vi "PPL_SIM_SIM_Execute.vi"(6 "FPGA_Time_Seconds":dbl, 8 "error in (no error)":errorcluster) -> (0 "error out":errorcluster)   [LabVIEW 2019]
uses:
  <vilib>/Rock Robotics/WPI/ThirdParty/JAS_Junk/TrajLib/Enum/DCMOTOR_TYPES_ENUM.ctl
  <vilib>/Rock Robotics/WPI/ThirdParty/JAS_Junk/TrajLib/Enum/DIFF_DRIVE_ToughBoxMini_GearChoice_ENUM.ctl
  <vilib>/Rock Robotics/WPI/ThirdParty/JAS_Junk/TrajLib/Enum/DIFF_DRIVE_TRAIN_SIM_STATE_ENUM.ctl
  <vilib>/Rock Robotics/WPI/ThirdParty/JAS_Junk/TrajLib/Rotation2d_CreateAngle.vi
  <vilib>/Rock Robotics/WPI/ThirdParty/JAS_Junk/TrajLib/Translation2d_Create.vi
  <vilib>/Rock Robotics/WPI/ThirdParty/JAS_Junk/TrajLib/BatterySim_CalculateLoadedBatteryVoltage.vi
  PPL_SIM_SIM_Globals.vi
  <vilib>/Rock Robotics/WPI/ThirdParty/JAS_Junk/TrajLib/Trajectory_Library.lvlib
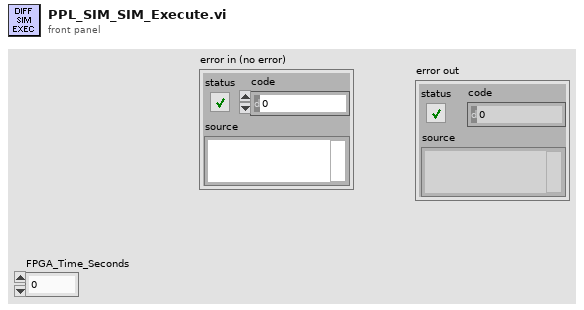
[diagram p1: front panel]
types:
  T1 = typedef "Trajectory_Library.lvlib/DIFF_DRIVE_TRAIN_SIM_STATE_ENUM.ctl" = enum16{"X_POS", "Y_POS", "HEADING", "LEFT_VEL", "RIGHT_VEL", "LEFT_DIST", "RIGHT_DIST"}
  T2 = typedef "Trajectory_Library.lvlib/DIFF_DRIVE_ToughBoxMini_GearChoice_ENUM.ctl" = enum16{"Ratio_12_75", "Ratio_10_71", "Ratio_8_45", "Ratio_7_31", "Ratio_5_95"}
  T3 = typedef "Trajectory_Library.lvlib/DCMOTOR_TYPES_ENUM.ctl" = enum16{"CIM", "AndyMark 9015", "Andy Mark RS 775 125", "Bag", "BaneBots RS 550", "BaneBots RS 775", "Falcon 500", "Mini CIM", "NEO", "NEO 550", "Romi BuiltIn", "Vex 775 Pro", "Snow Blower AM 2235A", "Bosch Seat AM 3493"}
  T4 = cluster{"Diff Motor Device Index":i32, "Wheel Encoder Device Index":i32, "Wheel DistPerzcount":dbl}[]
  T5 = cluster{"Diff Motor Device Index":i32, "Wheel Encoder Device Index":i32, "Wheel DistPerzcount":dbl}
  T6 = typedef "Trajectory_Library.lvlib/POSE2D.ctl" = cluster{"TRANSLATION":T7, "ROTATION":T8}
  T7 = typedef "Trajectory_Library.lvlib/TRANSLATION2D.ctl" = cluster{"X":dbl, "Y":dbl}
  T8 = typedef "Trajectory_Library.lvlib/ROTATION2D.ctl" = cluster{"VALUE":dbl, "COS":dbl, "SIN":dbl}
  T9 = typedef "Trajectory_Library.lvlib/DIFF_DRIVE_ODOM2.ctl" = cluster{"M_POSE_Meters":T6, "M_GyroOffset":T8, "M_PrevAngle":T8, "M_PrevLeftDist_M":dbl, "M_PrevRightDist_M":dbl, "M_InitLeftDist_M":dbl, "M_InitRightDist_M":dbl}
  T10 = typedef "Trajectory_Library.lvlib/DIFF_DRIVE_SIM_SIMULATION_PARAMS.ctl" = cluster{"X Pos Meas Std Dev M":dbl, "Y Pos Meas Std Dev M":dbl, "Heading Meas Std Dev Rad":dbl, "Left Vel Meas Std Dev M/S":dbl, "Right Vel Meas Std Dev M/S":dbl, "Left Pos Meas Std Dev M":dbl, "Right Pos Meas Std Dev M":dbl}
  T11 = typedef "Trajectory_Library.lvlib/DIFF_DRIVE_SIM_MODEL_PARAMS.CTL" = cluster{"TracWidth_M":dbl, "WheelRadius_M":dbl, "Gearing":dbl, "Mass kg":dbl, "MOI kgm2":dbl, "DCMOTOR_TYPES":T3, "Num Motors":i32}
  T12 = typedef "Trajectory_Library.lvlib/DIFF_DRIVE_TRAIN_SIM.ctl" = cluster{"m_Plant":T13, "m_X":T14, "m_Y":T14, "m_U":T14, "MeasureStdDev":T14, "m_Motor":T15, "m_OriginalGearing":dbl, "m_CurrentGearing":dbl, "m_WheelRadius_M":dbl, "m_RB":dbl}
  T13 = typedef "Trajectory_Library.lvlib/LINEAR_SYSTEM.ctl" = cluster{"m_A":T14, "m_B":T14, "m_C":T14, "m_D":T14, "States":i32, "Inputs":i32, "Outputs":i32}
  T14 = typedef "NI_Matrix.lvlib/RealMatrix.ctl" = dbl[][]
  T15 = typedef "Trajectory_Library.lvlib/DCMOTOR.CTL" = cluster{"nominalVoltage_Volts":dbl, "StallTorque_NM":dbl, "StallCurrent_Amps":dbl, "FreeCurrent_Amps":dbl, "FreeSpeed_RadPerSec":dbl, "R_Ohms":dbl, "KvINV_RadPerSecPerVolt":dbl, "Kt_NMPerAmp":dbl, "L_H":dbl, "Jr_KgM2":dbl}
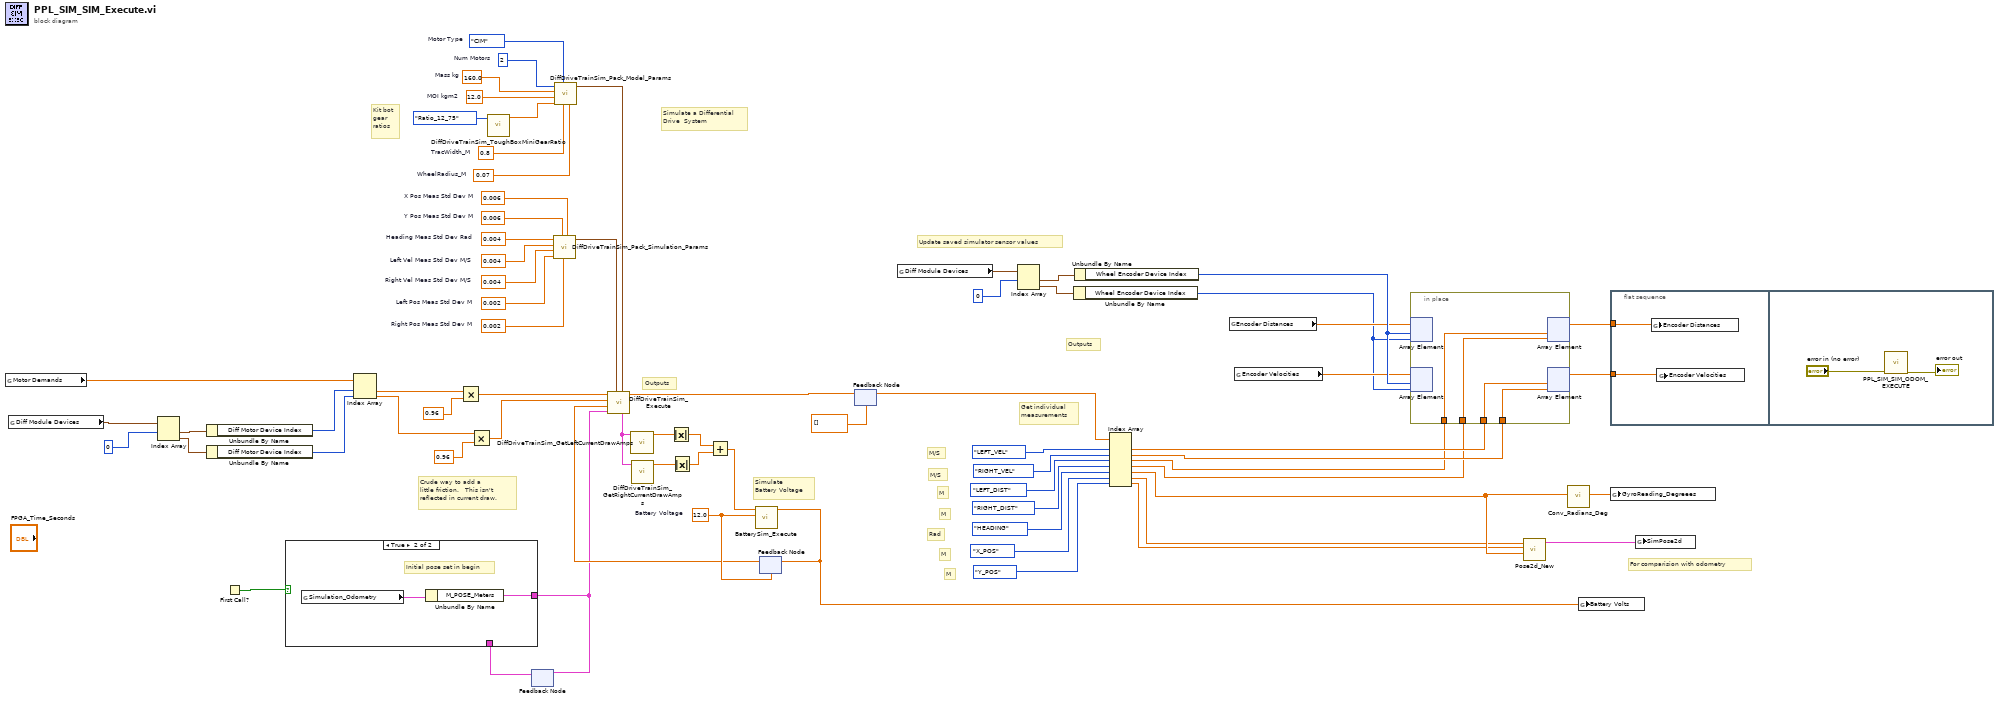
[diagram p0: block diagram]
diagram:
  w57 = 160.0  # Mass kg
  w58 = 12.0  # MOI kgm2
  w59 = 0.8  # TracWidth_M
  w60 = 0.07  # WheelRadius_M
  w61 = 0.004  # Heading Meas Std Dev Rad
  w62 = 0.004  # Left Vel Meas Std Dev M/S
  w63 = 0.004  # Right Vel Meas Std Dev M/S
  w64 = 0.002  # Left Pos Meas Std Dev M
  w65 = 0.006  # Y Pos Meas Std Dev M
  w66 = 0.002  # Right Pos Meas Std Dev M
  w67 = 0.006  # X Pos Meas Std Dev M
  w70 = 2  # Num Motors
  w71 = DCMOTOR_TYPES_ENUM."CIM"  # Motor Type
  w47 = 12.0  # Battery Voltage
  # "For comparision with odometry"
  # "M"
  # "M"
  # "Rad"
  # "M"
  # "M"
  # "M/S"
  # "M/S"
  # "Update saved simulator sensor values"
  # "Crude way to add a \nlittle friction.   This isn't\nreflected in current draw."
  # "Get individual\nmeasurements"
  # "Kit bot\ngear \nratios"
  # "Outputs"
  # "Simulate\nBattery Voltage"
  # "Simulate a Differential\nDrive  System"
  # "Outputs"
  n1 = global read "PPL_SIM_SIM_Globals.vi" "Motor Demands"() -> (w39:dbl[])
  n2 = global read "PPL_SIM_SIM_Globals.vi" "Diff Module Devices"() -> (w41:T4)
  n3 = Index Array(array=w41, index #1=0 ("Module Index")) -> (element #1=w40:T5, element #2=w34:T5)  [unwired: 1 in]
  n4 = Unbundle By Name(w40) -> ("Diff Motor Device Index"=w38:i32)
  n5 = Unbundle By Name(w34) -> ("Diff Motor Device Index"=w33:i32)
  n6 = First Call?() -> (First Call?: T/F=w7:bool)
  n7 = Index Array(array=w39, index #1=w38, index #2=w33) -> (element #1=w35:dbl, element #2=w31:dbl)
  n8 = Multiply(x=w35, y=0.96) -> (x*y=w30:dbl)
  n9 = Multiply(x=w31, y=0.96) -> (x*y=w22:dbl)
  n10 = call <vilib>:"DiffDriveTrainSim_ToughBoxMiniGearRatio.vi"("ToughBoxMiniGear"=DIFF_DRIVE_ToughBoxMini_GearChoice_ENUM."Ratio_12_75") -> ("GearRatio"=w55:dbl)  [unwired: 10 in]
  n11 = feedback #1() -> (w5:T6)  [unwired: 1 in]
  n12 = case shown="True" w7 {
    tunnel: [w72 w73] -> w6
    tunnel: w5 -> [w72 _]
    frame False {
    }
    frame True {
      # "Initial pose set in begin"
      n13 = global read "PPL_SIM_SIM_Globals.vi" "Simulation_Odometry"() -> (w74:T9)
      n14 = Unbundle By Name(w74) -> ("M_POSE_Meters"=w73:T6)
    }
  }
  n15 = feedback-in #1(w6) -> ()
  n16 = call <vilib>:"DiffDriveTrainSim_Pack_Simulation_Params.vi"("X Pos Meas Std Dev M"=w67, "Right Pos Meas Std Dev M"=w66, "Y Pos Meas Std Dev M"=w65, "Left Pos Meas Std Dev M"=w64, "Right Vel Meas Std Dev M/S"=w63, "Left Vel Meas Std Dev M/S"=w62, "Heading Meas Std Dev Rad"=w61) -> ("DiffDriveSim_Simulation _Params"=w68:T10)  [unwired: 4 in]
  n17 = call <vilib>:"DiffDriveTrainSim_Pack_Model_Params.vi"("WheelRadius_M"=w60, "TracWidth_M"=w59, "DCMOTOR_TYPES"=w71, "Gearing"=w55, "MOI kgm2"=w58, "Mass kg"=w57, "Num Motors"=w70) -> ("DiffDriveSim_Model _Params"=w69:T11)  [unwired: 4 in]
  n18 = feedback #2(w47) -> (w46:dbl)
  n19 = call <vilib>:"DiffDriveTrainSim_Execute.vi"("LinearSystem_ID_DiffDrv_Model"=w69, "DiffDriveSim_Simulation _Params"=w68, "Initial Pose"=w6, "BatteryVoltage"=w46, "Right Motor Dmd"=w22, "Left Motor Dmd"=w30) -> ("Outputs"=w45:dbl[], "out DiffDriveTrainSim"=w54:T12)  [unwired: 3 in, 1 out]
  n20 = call <vilib>:"DiffDriveTrainSim_GetLeftCurrentDrawAmps.vi"("DiffDriveTrainSim"=w54) -> ("LeftCurrentDraw_Amps"=w25:dbl)  [unwired: 10 in]
  n21 = call <vilib>:"DiffDriveTrainSim_GetRightCurrentDrawAmps.vi"("DiffDriveTrainSim"=w54) -> ("RightCurrentDraw_Amps"=w26:dbl)  [unwired: 10 in]
  n22 = Absolute Value(x=w25) -> (abs(x)=w24:dbl)
  n23 = Absolute Value(x=w26) -> (abs(x)=w23:dbl)
  n24 = Add(x=w24, y=w23) -> (x+y=w53:dbl)
  n25 = call <vilib>:"BatterySim_Execute.vi"("Nominal Battery Voltage"=w47, "Current"=w53) -> ("Voltage"=w27:dbl)  [unwired: 9 in]
  n26 = feedback-in #2(w27) -> ()
  n27 = feedback #3(dbl[] [] ("Outputs")) -> (w44:dbl[])
  n28 = feedback-in #3(w45) -> ()
  n29 = global read "PPL_SIM_SIM_Globals.vi" "Diff Module Devices"() -> (w21:T4)
  n30 = Index Array(array=w21, index #1=0 ("index")) -> (element #1=w20:T5, element #2=w15:T5)  [unwired: 1 in]
  n31 = Unbundle By Name(w15) -> ("Wheel Encoder Device Index"=w14:i32)
  n32 = Unbundle By Name(w20) -> ("Wheel Encoder Device Index"=w19:i32)
  n33 = Index Array(array=w44, index #1=DIFF_DRIVE_TRAIN_SIM_STATE_ENUM."LEFT_VEL" ("DIFF_DRIVE_TRAIN_SIM_STATE"), index #2=DIFF_DRIVE_TRAIN_SIM_STATE_ENUM."RIGHT_VEL" ("DIFF_DRIVE_TRAIN_SIM_STATE"), index #3=DIFF_DRIVE_TRAIN_SIM_STATE_ENUM."LEFT_DIST" ("DIFF_DRIVE_TRAIN_SIM_STATE"), index #4=DIFF_DRIVE_TRAIN_SIM_STATE_ENUM."RIGHT_DIST" ("DIFF_DRIVE_TRAIN_SIM_STATE"), index #5=DIFF_DRIVE_TRAIN_SIM_STATE_ENUM."HEADING" ("DIFF_DRIVE_TRAIN_SIM_STATE"), index #6=DIFF_DRIVE_TRAIN_SIM_STATE_ENUM."X_POS" ("DIFF_DRIVE_TRAIN_SIM_STATE"), index #7=DIFF_DRIVE_TRAIN_SIM_STATE_ENUM."Y_POS" ("DIFF_DRIVE_TRAIN_SIM_STATE")) -> (element #1=w13:dbl, element #2=w12:dbl, element #3=w11:dbl, element #4=w10:dbl, element #5=w4:dbl, element #6=w3:dbl, element #7=w2:dbl)
  n34 = global read "PPL_SIM_SIM_Globals.vi" "Encoder Distances"() -> (w18:dbl[])
  n35 = global read "PPL_SIM_SIM_Globals.vi" "Encoder Velocities"() -> (w17:dbl[])
  n36 = in-place {
    in-place-border: w11 -> [w77]
    in-place-border: w13 -> [w78]
    in-place-border: w12 -> [w76]
    in-place-border: w10 -> [w75]
    n37 = in-place-array #4(w18, w19, w14) -> ()  [unwired: 2 out]
    n38 = in-place-array #5(w17, w19, w14) -> ()  [unwired: 2 out]
    n39 = in-place-array #4(w77, w75) -> (w8:dbl[])  [unwired: 2 out]
    n40 = in-place-array #5(w78, w76) -> (w9:dbl[])  [unwired: 2 out]
  }
  n41 = call <vilib>:"Pose2d_New.vi"("Heading"=w4, "Y"=w2, "X"=w3) -> ("out POSe"=w1:T6)  [unwired: 8 in]
  n42 = call <vilib>:"Conv_Radians_Deg.vi"("Radians"=w4) -> ("Degrees"=w42:dbl)  [unwired: 10 in]
  n43 = global write "PPL_SIM_SIM_Globals.vi" "Battery Volts"(w27) -> ()
  n44 = flat-sequence {
    tunnel: w9 -> [w80]
    tunnel: w8 -> [w79]
    frame #0 {
      n45 = global write "PPL_SIM_SIM_Globals.vi" "Encoder Distances"(w79) -> ()
      n46 = global write "PPL_SIM_SIM_Globals.vi" "Encoder Velocities"(w80) -> ()
    }
    frame #1 {
      n47 = call "PPL_SIM_SIM_ODOM_EXECUTE.vi"("error in (no error)"="error in (no error)") -> ("error out"=→"error out":errorcluster)  [unwired: 10 in]
    }
  }
  n48 = global write "PPL_SIM_SIM_Globals.vi" "GyroReading_Degreees"(w42) -> ()
  n49 = global write "PPL_SIM_SIM_Globals.vi" "SimPose2d"(w1) -> ()
